vi "Error Code to Error Cluster.vi"(7 "Error Code":i32, 13 "Error In":errorcluster) -> (2 "Error Out":errorcluster)   [LabVIEW 2019]
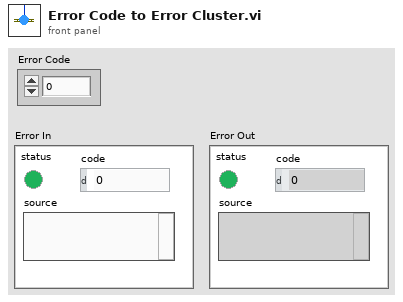
[diagram p1: front panel]
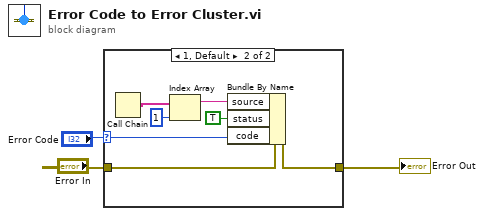
[diagram p0: block diagram]
diagram:
  n1 = case shown="1, Default" "Error Code" {
    selector: "Error Code" -> [_ w9]
    tunnel: "Error In" -> [w4 w11]
    tunnel: [w4 w10] -> w1
    frame 0 {
    }
    frame 1, Default {
      n2 = Call Chain() -> (call chain=w7:string[])
      n3 = Index Array(array=w7, index=1) -> (element=w6:string)
      n4 = Bundle By Name(cluster=w11, "source"=w6, "status"=TRUE, "code"=w9) -> (w10:errorcluster)
    }
  }
  "Error Out" <- w1
